vi "AWG Set and Arm.vi"(7 "pulse count (0: infinite)":i32, 8 "error in (no error)":errorcluster, 9 "trigger":T1, 10 "sampling rate":T5, 11 "awg session in":T7={"type"=enum."Agilent 331xxA to 332xxA", "VISA"="", "enable 10MHz ref"=FALSE, "cmi ckd2"={"VISA"="", "clock source"=enum."Auto", "manual ref clk"=FALSE, "ref clock [Hz]"=0.0}, "cmi sync v3"={"VISA"="", "baud rate [bd/s]"=115200, "source"=enum."Auto", "hv range"=enum."1kV", "fsrc is fixed"=FALSE, "fsrc [Hz]"=10000000.0, "freq integ [s]"=1.0, "freq filter"=5, "trig level"=enum."TTL 5V", "chn1 mode"=enum."Source divider", "chn1 level"=enum."Positive 5V", "chn2 mode"=enum."Source divider", "chn2 level"=enum."Positive 5V", "chn2 div"=1, "chn3 mode"=enum."Chn 1 Active", "chn3 level"=enum."Positive 5V", "chn1 div entry"=enum."Calculate nearest divisor from measured fx", "chn1 dev limit [%]"=1.0, "chn1 check dev"=FALSE}, "trigger"={"source"=enum."Immediate", "level [V]"=0.0, "coupling"=enum."DC", "slope"=enum."POS"}} {"cmi sync v3"."chn2 div" min=1 max=100000000 step=1; "cmi sync v3"."fsrc [Hz]" format="%_8p"}) -> (0 "error out":errorcluster, 3 "awg session out":T7={"type"=enum."Agilent 331xxA to 332xxA", "VISA"="", "enable 10MHz ref"=FALSE, "cmi ckd2"={"VISA"="", "clock source"=enum."Auto", "manual ref clk"=FALSE, "ref clock [Hz]"=0.0}, "cmi sync v3"={"VISA"="", "baud rate [bd/s]"=115200, "source"=enum."Auto", "hv range"=enum."1kV", "fsrc is fixed"=FALSE, "fsrc [Hz]"=10000000.0, "freq integ [s]"=1.0, "freq filter"=5, "trig level"=enum."TTL 5V", "chn1 mode"=enum."Source divider", "chn1 level"=enum."Positive 5V", "chn2 mode"=enum."Source divider", "chn2 level"=enum."Positive 5V", "chn2 div"=1, "chn3 mode"=enum."Chn 1 Active", "chn3 level"=enum."Positive 5V", "chn1 div entry"=enum."Calculate nearest divisor from measured fx", "chn1 dev limit [%]"=1.0, "chn1 check dev"=FALSE}, "trigger"={"source"=enum."Immediate", "level [V]"=0.0, "coupling"=enum."DC", "slope"=enum."POS"}} {"cmi sync v3"."chn2 div" min=1 max=100000000 step=1; "cmi sync v3"."fsrc [Hz]" format="%_8p"})   [LabVIEW 2020, in "AWG.lvlib"]
doc: "AWG wrapper: This sets the AWG to desired frequency and arms it. No pulses are generated here. Waiting for trigger!"
uses:
  AWG.lvlib
  AWG Session.ctl
  AWG Type.ctl
  CMI Clock Divider v2/CMI ckd2 Session.ctl
  CMI Clock Divider v2/CMI ckd2 Source Mode.ctl
  CMI Sync V3/CMI Sync V3 session.ctl
  CMI Sync V3/Configure/CMI Sync V3 Reference Clock Source.ctl
  CMI Sync V3/Configure/CMI Sync V3 HV input Range.ctl
  CMI Sync V3/Configure/CMI Sync V3 Trigger Input Level.ctl
  CMI Sync V3/Configure/CMI Sync V3 Channel 1 Mode.ctl
  CMI Sync V3/Configure/CMI Sync V3 Channel Output Levels.ctl
  CMI Sync V3/Configure/CMI Sync V3 Channel 2 Mode.ctl
  CMI Sync V3/Configure/CMI Sync V3 Channel 3 Mode.ctl
  adc/ADC Trig Config.ctl
  adc/ADC Trig Mode Source.ctl
  adc/ADC Trig Coupling.ctl
  adc/ADC Trig Slope.ctl
  DMM/3458A Sampling Rate.ctl
  AWG Clock Setup Mode.ctl
  Agilent 33XXX Series/Agilent 33XXX Series.lvlib
  AFG3000/Tektronix AFG 3000 Series.lvlib
  CMI Sync V3/CMI Sync Unit V3.lvlib
  DMM/3458A Virtual Digitizer.lvlib
  CMI Sync V3/Configure/CMI Sync V3 Channel 1 Divisor Entry Mode.ctl
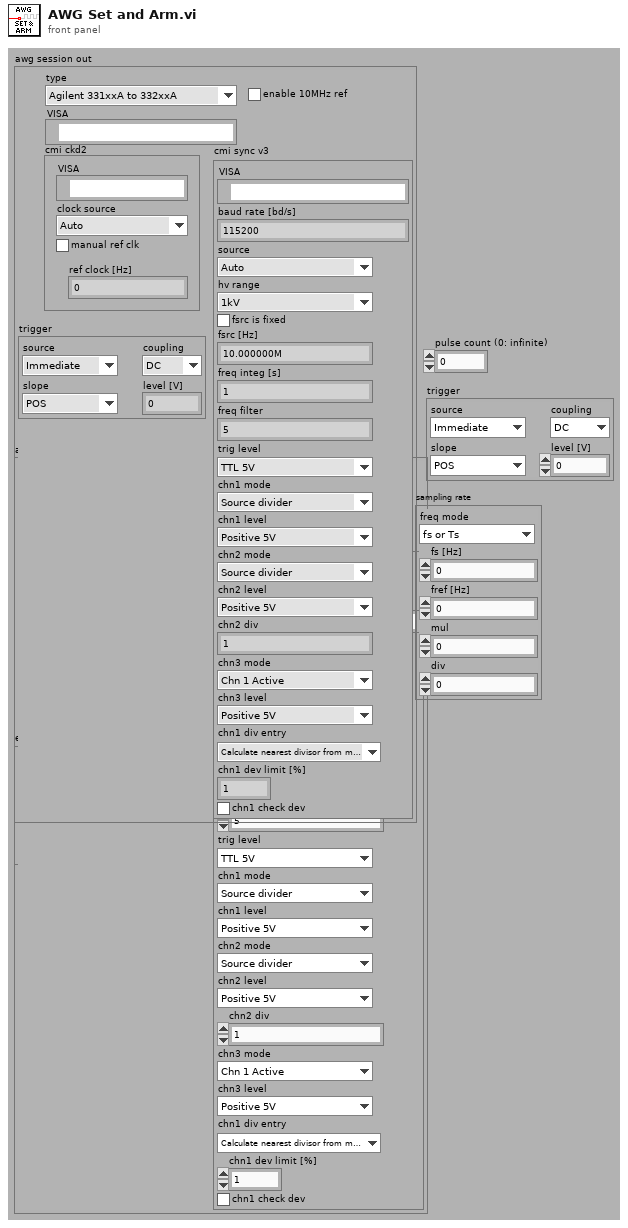
[diagram p1: front panel]
types:
  T1 = typedef "ADC Trig Config.ctl" = cluster{"source":T2, "level [V]":dbl, "coupling":T3, "slope":T4}
  T2 = typedef "ADC Trig Mode Source.ctl" = enum16{"Immediate", "External", "Level"}
  T3 = typedef "ADC Trig Coupling.ctl" = enum16{"DC", "AC"}
  T4 = typedef "ADC Trig Slope.ctl" = enum16{"POS", "NEG"}
  T5 = typedef "3458A Virtual Digitizer.lvlib/3458A Sampling Rate.ctl" = cluster{"freq mode":T6, "fs [Hz]":dbl, "fref [Hz]":dbl, "mul":dbl, "div":dbl}
  T6 = typedef "AWG.lvlib/AWG Clock Setup Mode.ctl" = enum16{"fs or Ts", "fs or Ts with fref", "fref/N", "fref*M/N", "fref*Ratio"}
  T7 = typedef "AWG.lvlib/AWG Session.ctl" = cluster{"type":T8, "VISA":refnum<visa-resource-name>, "enable 10MHz ref":bool, "cmi ckd2":T9, "cmi sync v3":T11, "trigger":T1}
  T8 = typedef "AWG.lvlib/AWG Type.ctl" = enum16{"Agilent 331xxA to 332xxA", "Agilent 335xxA to 336xxA", "Tektronix AFG3101C", "CMI Clock Divider v2", "CMI Sync Unit V3", "dummy"}
  T9 = typedef "AWG.lvlib/CMI ckd2 Session.ctl" = cluster{"VISA":refnum<visa-resource-name>, "clock source":T10, "manual ref clk":bool, "ref clock [Hz]":dbl}
  T10 = typedef "AWG.lvlib/CMI ckd2 Source Mode.ctl" = enum16{"Auto", "LF clock", "HF clock", "Internal"}
  T11 = typedef "AWG.lvlib/CMI Sync Unit V3.lvlib/CMI Sync V3 session.ctl" = cluster{"VISA":refnum<visa-resource-name>, "baud rate [bd/s]":i32, "source":T12, "hv range":T13, "fsrc is fixed":bool, "fsrc [Hz]":dbl, "freq integ [s]":dbl, "freq filter":i32, "trig level":T14, "chn1 mode":T15, "chn1 level":T16, "chn2 mode":T17, "chn2 level":T16, "chn2 div":i32, "chn3 mode":T18, "chn3 level":T16, "chn1 div entry":T19, "chn1 dev limit [%]":dbl, "chn1 check dev":bool}
  T12 = typedef "AWG.lvlib/CMI Sync Unit V3.lvlib/CMI Sync V3 Reference Clock Source.ctl" = enum16{"Auto", "Internal", "Logic", "Sine", "HV"}
  T13 = typedef "AWG.lvlib/CMI Sync Unit V3.lvlib/CMI Sync V3 HV input Range.ctl" = enum16{"10V", "60V", "250V", "1kV"}
  T14 = typedef "AWG.lvlib/CMI Sync Unit V3.lvlib/CMI Sync V3 Trigger Input Level.ctl" = enum16{"LVCMOS 3V3", "TTL 5V"}
  T15 = typedef "AWG.lvlib/CMI Sync Unit V3.lvlib/CMI Sync V3 Channel 1 Mode.ctl" = enum16{"Source divider", "DDS absolute", "DDS ratio", "DDS ratio M/N"}
  T16 = typedef "AWG.lvlib/CMI Sync Unit V3.lvlib/CMI Sync V3 Channel Output Levels.ctl" = enum16{"Positive 3V3", "Negative 3V3", "Positive 5V", "Negative 5V"}
  T17 = typedef "AWG.lvlib/CMI Sync Unit V3.lvlib/CMI Sync V3 Channel 2 Mode.ctl" = enum16{"Source divider", "Chn 1 divide"}
  T18 = typedef "AWG.lvlib/CMI Sync Unit V3.lvlib/CMI Sync V3 Channel 3 Mode.ctl" = enum16{"Chn 1 Active", "Chn 2 Active", "Chn 1 Trigger", "Chn 2 Trigger", "Gate", "PPS", "10MHz"}
  T19 = typedef "AWG.lvlib/CMI Sync Unit V3.lvlib/CMI Sync V3 Channel 1 Divisor Entry Mode.ctl" = enum16{"Set divisor directly", "Calculate nearest divisor from measured fx"}
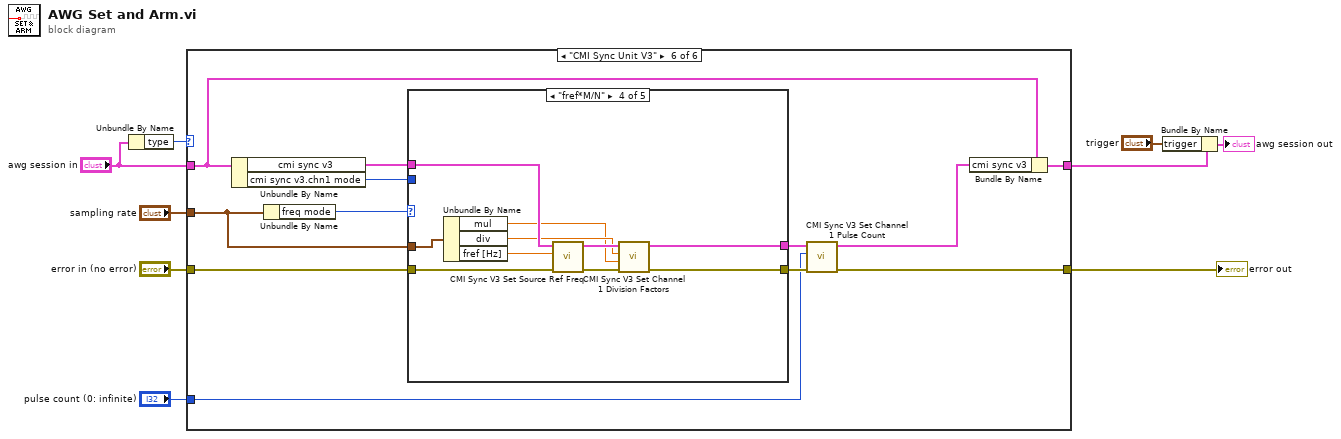
[diagram p0: block diagram]
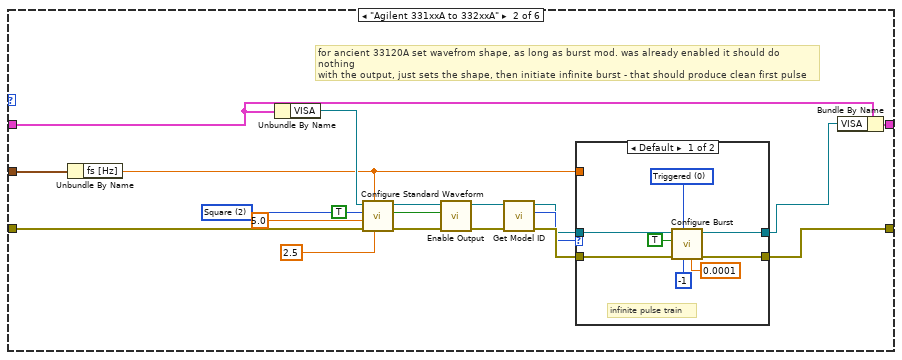
[diagram p3: hidden frame]
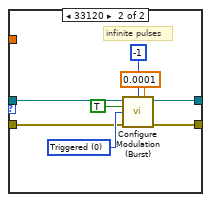
[diagram p4: hidden frame]
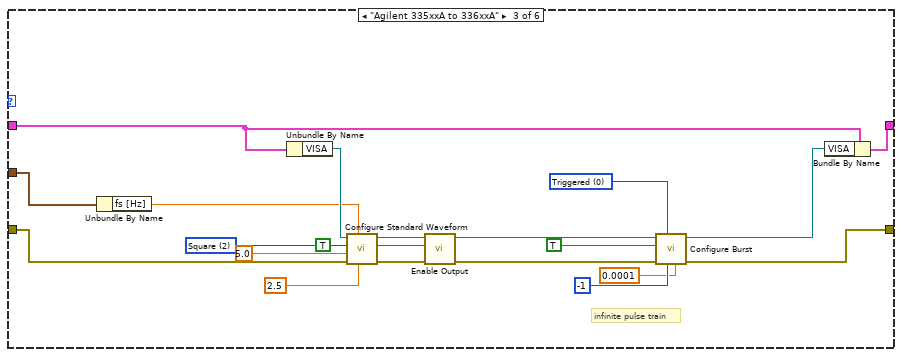
[diagram p5: hidden frame]
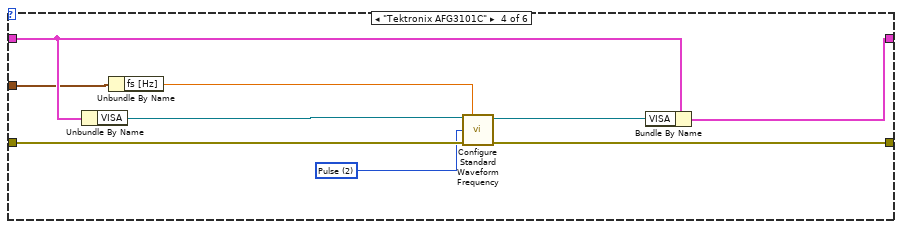
[diagram p6: hidden frame]
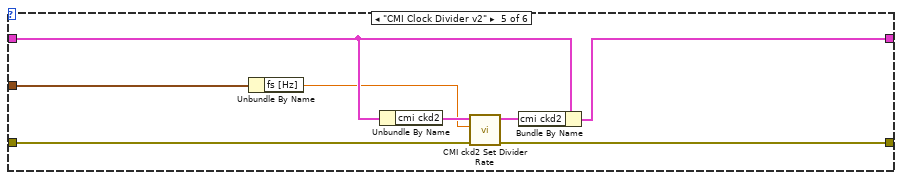
[diagram p7: hidden frame]
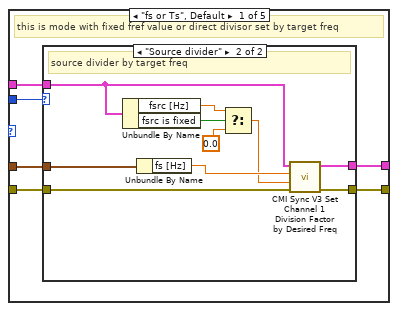
[diagram p8: hidden frame]
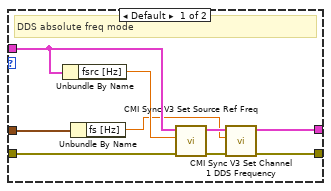
[diagram p9: hidden frame]
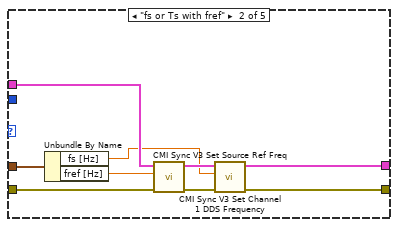
[diagram p10: hidden frame]
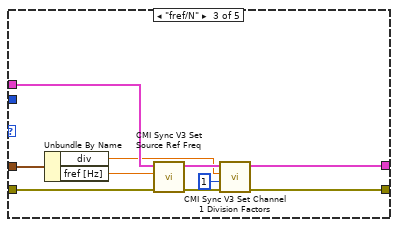
[diagram p11: hidden frame]
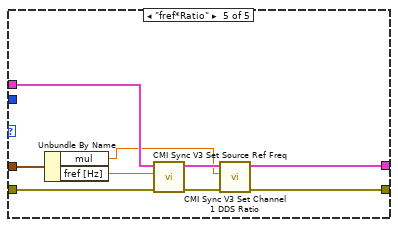
[diagram p12: hidden frame]
diagram:
  n1 = Unbundle By Name("awg session in") -> ("type"=w9:T8)
  n2 = case shown="\"CMI Sync Unit V3\"" w9 {
    tunnel: "error in (no error)" -> [w11 w25 w56 w72 w83 w94]
    tunnel: [w11 w14 w49 w69 w78 w88] -> w7
    tunnel: "awg session in" -> [w10 w29 w66 w75 w81 w90]
    tunnel: [w10 w30 w65 w74 w77 w91] -> w4
    tunnel: "sampling rate" -> [_ w15 w57 w68 w79 w92]
    tunnel: "pulse count (0: infinite)" -> [_ _ _ _ _ w87]
    frame Default {
    }
    frame "Agilent 331xxA to 332xxA" {
      w28 = u16 2 items=["DC", "Sine", "Square", "Triangle", "Ramp", "Pulse", "Noise", "Sinc", "Negative Ramp", "Exponential Rise", "Exponential Fall", "Cardiac"] ("Waveform Function (1: Sine)")
      # "for ancient 33120A set wavefrom shape, as long as burst mod. was already enabled it should do nothing\nwith the output, just sets the shape, then initiate infinite burst - that should produce clean first pulse"
      n3 = Unbundle By Name(w15) -> ("fs [Hz]"=w12:dbl)
      n4 = Unbundle By Name(w29) -> ("VISA"=w26:refnum<visa-resource-name>)
      n5 = call "Configure Standard Waveform.vi"("DC Offset (0.00 V)"=2.5, "Frequency (1000 Hz)"=w12, "error in (no error)"=w25, "Amplitude (1)"=5.0, "Waveform Function (1: Sine)"=w28, "VISA resource name"=w26) -> ("error out"=w23:errorcluster, "VISA resource name out"=w22:refnum<visa-resource-name>)  [unwired: 4 in]
      n6 = call "Enable Output.vi"("error in (no error)"=w23, "Enable Output  (T: Enable)"=TRUE, "VISA resource name"=w22) -> ("error out"=w20:errorcluster, "VISA resource name out"=w19:refnum<visa-resource-name>)  [unwired: 7 in]
      n7 = call "Get Model ID.vi"("error in (no error)"=w20, "VISA resource name"=w19) -> ("error out"=w18:errorcluster, "model ID"=w17:u32, "VISA resource name out"=w16:refnum<visa-resource-name>)  [unwired: 7 in]
      n8 = case shown="Default" w17 {
        tunnel: [w37 w43] -> w14
        tunnel: [w36 w42] -> w13
        tunnel: w12 -> [_ _]
        tunnel: w18 -> [w38 w41]
        tunnel: w16 -> [w35 w40]
        frame Default {
          w34 = u16 0 items=["Triggered", "Gated"] ("Burst Mode (0: Triggered)")
          # "infinite pulse train"
          n9 = call "Configure Burst.vi"("Burst Period (1 s)"=0.0001, "Burst Count (1)"=-1, "Burst Mode (0: Triggered)"=w34, "error in (no error)"=w38, "Enable Burst (T: Enable)"=TRUE, "VISA resource name"=w35) -> ("error out"=w37:errorcluster, "VISA resource name out"=w36:refnum<visa-resource-name>)  [unwired: 4 in]
        }
        frame 33120 {
          w44 = u16 0 items=["Triggered", "Gated"] ("Burst Modulation Mode (0: Triggered)")
          # "infinite pulses"
          n10 = call "Configure Modulation (Burst).vi"("VISA resource name"=w40, "Burst Count (1)"=-1, "Burst Period (1 s)"=0.0001, "Enable Burst Modulation (T: Enable)"=TRUE, "Burst Modulation Mode (0: Triggered)"=w44, "error in (no error)"=w41) -> ("VISA resource name out"=w42:refnum<visa-resource-name>, "error out"=w43:errorcluster)  [unwired: 8 in]
        }
      }
      n11 = Bundle By Name(cluster=w29, "VISA"=w13) -> (w30:T7)
    }
    frame "Agilent 335xxA to 336xxA" {
      w55 = u16 0 items=["Triggered", "Gated"] ("Burst Mode (0: Triggered)")
      w64 = u16 2 items=["DC", "Sine", "Square", "Triangle", "Ramp", "Pulse", "Noise", "Sinc", "Negative Ramp", "Exponential Rise", "Exponential Fall", "Cardiac"] ("Waveform Function (1: Sine)")
      # "infinite pulse train"
      n12 = Unbundle By Name(w57) -> ("fs [Hz]"=w47:dbl)
      n13 = Unbundle By Name(w66) -> ("VISA"=w58:refnum<visa-resource-name>)
      n14 = call "Configure Standard Waveform.vi"("DC Offset (0.00 V)"=2.5, "Frequency (1000 Hz)"=w47, "error in (no error)"=w56, "Amplitude (1)"=5.0, "Waveform Function (1: Sine)"=w64, "VISA resource name"=w58) -> ("error out"=w61:errorcluster, "VISA resource name out"=w60:refnum<visa-resource-name>)  [unwired: 4 in]
      n15 = call "Enable Output.vi"("error in (no error)"=w61, "Enable Output  (T: Enable)"=TRUE, "VISA resource name"=w60) -> ("error out"=w51:errorcluster, "VISA resource name out"=w50:refnum<visa-resource-name>)  [unwired: 7 in]
      n16 = call "Configure Burst.vi"("Burst Period (1 s)"=0.0001, "Burst Count (1)"=-1, "Burst Mode (0: Triggered)"=w55, "error in (no error)"=w51, "Enable Burst (T: Enable)"=TRUE, "VISA resource name"=w50) -> ("error out"=w49:errorcluster, "VISA resource name out"=w48:refnum<visa-resource-name>)  [unwired: 4 in]
      n17 = Bundle By Name(cluster=w66, "VISA"=w48) -> (w65:T7)
    }
    frame "Tektronix AFG3101C" {
      w71 = u16 2 items=["Sine", "Square", "Pulse", "Ramp", "Noise", "DC", "Sin(x)/x", "Gaussian", "Lorentz", "Exponential Rise", "Exponential Decay", "Haversine"] ("Waveform Function (0: Sine)")
      n18 = Unbundle By Name(w75) -> ("VISA"=w73:refnum<visa-resource-name>)
      n19 = Unbundle By Name(w68) -> ("fs [Hz]"=w67:dbl)
      n20 = call "Configure Standard Waveform Frequency.vi"("VISA resource name"=w73, "Frequency (1000 Hz)"=w67, "Waveform Function (0: Sine)"=w71, "error in (no error)"=w72) -> ("VISA resource name out"=w70:refnum<visa-resource-name>, "error out"=w69:errorcluster)  [unwired: 10 in]
      n21 = Bundle By Name(cluster=w75, "VISA"=w70) -> (w74:T7)
    }
    frame "CMI Clock Divider v2" {
      n22 = Unbundle By Name(w79) -> ("fs [Hz]"=w76:dbl)
      n23 = Unbundle By Name(w81) -> ("cmi ckd2"=w82:T9)
      n24 = call "CMI ckd2 Set Divider Rate.vi"("error in"=w83, "clock rate [Hz]"=w76, "session"=w82) -> ("error out"=w78:errorcluster, "session out"=w80:T9)  [unwired: 6 in, 1 out]
      n25 = Bundle By Name(cluster=w81, "cmi ckd2"=w80) -> (w77:T7)
    }
    frame "CMI Sync Unit V3" {
      n26 = Unbundle By Name(w90) -> ("cmi sync v3"=w93:T11, "cmi sync v3.chn1 mode"=w84:T15)
      n27 = Unbundle By Name(w92) -> ("freq mode"=w95:T6)
      n28 = case shown="\"fref*M/N\"" w95 {
        tunnel: w94 -> [w101 w129 w139 w149 w158]
        tunnel: w93 -> [w97 w128 w138 w148 w157]
        tunnel: w92 -> [w100 w126 w136 w146 w155]
        tunnel: [w99 w123 w133 w143 w152] -> w89
        tunnel: [w98 w122 w132 w142 w151] -> w86
        tunnel: w84 -> [w96 _ _ _ _]
        frame "fs or Ts", Default {
          # "this is mode with fixed fref value or direct divisor set by target freq"
          n29 = case shown="\"Source divider\"" w96 {
            tunnel: w101 -> [w110 w120]
            tunnel: w100 -> [w108 w119]
            tunnel: [w106 w117] -> w99
            tunnel: [w105 w116] -> w98
            tunnel: w97 -> [w104 w115]
            frame Default {
              # "DDS absolute freq mode"
              n30 = Unbundle By Name(w104) -> ("fsrc [Hz]"=w103:dbl)
              n31 = Unbundle By Name(w108) -> ("fs [Hz]"=w102:dbl)
              n32 = call "CMI Sync V3 Set Source Ref Freq.vi"("error in"=w110, "Expected reference frequency [Hz]"=w103, "session in"=w104) -> ("error out"=w109:errorcluster, "session out"=w107:T11)  [unwired: 7 in]
              n33 = call "CMI Sync V3 Set Channel 1 DDS Frequency.vi"("error in"=w109, "DDS absolute [Hz] (1 MHz)"=w102, "session in"=w107) -> ("error out"=w106:errorcluster, "session out"=w105:T11)  [unwired: 7 in]
            }
            frame "Source divider" {
              # "source divider by target freq"
              n34 = Unbundle By Name(w115) -> ("fsrc [Hz]"=w113:dbl, "fsrc is fixed"=w114:bool)
              n35 = Unbundle By Name(w119) -> ("fs [Hz]"=w118:dbl)
              n36 = Select(t=w113, s=w114, f=0.0) -> (s? t:f=w111:dbl)
              n37 = call "CMI Sync V3 Set Channel 1 Division Factor by Desired Freq.vi"("error in"=w120, "explicit ref freq [Hz] (0: auto estimate)"=w111, "target output freq [Hz]"=w118, "session in"=w115) -> ("error out"=w117:errorcluster, "session out"=w116:T11)  [unwired: 4 in, 2 out]
            }
          }
        }
        frame "fs or Ts with fref" {
          n38 = Unbundle By Name(w126) -> ("fs [Hz]"=w121:dbl, "fref [Hz]"=w125:dbl)
          n39 = call "CMI Sync V3 Set Source Ref Freq.vi"("error in"=w129, "Expected reference frequency [Hz]"=w125, "session in"=w128) -> ("error out"=w127:errorcluster, "session out"=w124:T11)  [unwired: 7 in]
          n40 = call "CMI Sync V3 Set Channel 1 DDS Frequency.vi"("error in"=w127, "DDS absolute [Hz] (1 MHz)"=w121, "session in"=w124) -> ("error out"=w123:errorcluster, "session out"=w122:T11)  [unwired: 7 in]
        }
        frame "fref/N" {
          n41 = Unbundle By Name(w136) -> ("div"=w131:dbl, "fref [Hz]"=w135:dbl)
          n42 = call "CMI Sync V3 Set Source Ref Freq.vi"("error in"=w139, "Expected reference frequency [Hz]"=w135, "session in"=w138) -> ("error out"=w137:errorcluster, "session out"=w134:T11)  [unwired: 7 in]
          n43 = call "CMI Sync V3 Set Channel 1 Division Factors.vi"("error in"=w137, "DDS multiplier (1)"=1, "Divider (10)"=w131, "session in"=w134) -> ("error out"=w133:errorcluster, "session out"=w132:T11)  [unwired: 6 in]
        }
        frame "fref*M/N" {
          n44 = Unbundle By Name(w146) -> ("mul"=w140:dbl, "div"=w141:dbl, "fref [Hz]"=w145:dbl)
          n45 = call "CMI Sync V3 Set Source Ref Freq.vi"("error in"=w149, "Expected reference frequency [Hz]"=w145, "session in"=w148) -> ("error out"=w147:errorcluster, "session out"=w144:T11)  [unwired: 7 in]
          n46 = call "CMI Sync V3 Set Channel 1 Division Factors.vi"("error in"=w147, "DDS multiplier (1)"=w140, "Divider (10)"=w141, "session in"=w144) -> ("error out"=w143:errorcluster, "session out"=w142:T11)  [unwired: 6 in]
        }
        frame "fref*Ratio" {
          n47 = Unbundle By Name(w155) -> ("mul"=w150:dbl, "fref [Hz]"=w154:dbl)
          n48 = call "CMI Sync V3 Set Source Ref Freq.vi"("error in"=w158, "Expected reference frequency [Hz]"=w154, "session in"=w157) -> ("error out"=w156:errorcluster, "session out"=w153:T11)  [unwired: 7 in]
          n49 = call "CMI Sync V3 Set Channel 1 DDS Ratio.vi"("error in"=w156, "DDS ratio (1.0)"=w150, "session in"=w153) -> ("error out"=w152:errorcluster, "session out"=w151:T11)  [unwired: 7 in]
        }
      }
      n50 = call "CMI Sync V3 Set Channel 1 Pulse Count.vi"("error in"=w89, "Pulse count (0: infinite)"=w87, "session in"=w86) -> ("error out"=w88:errorcluster, "session out"=w85:T11)  [unwired: 7 in]
      n51 = Bundle By Name(cluster=w90, "cmi sync v3"=w85) -> (w91:T7)
    }
  }
  "error out" <- w7
  n52 = Bundle By Name(cluster=w4, "trigger"="trigger") -> (→"awg session out":T7)
